vi "UpdateConfigInInternal.vi"(2 "error in (no error)":errorcluster, 3 "IntTime":i32, 4 "Instruments in":refnum<class "Instruments.lvclass">) -> (0 "error out":errorcluster, 1 "Instruments out":refnum<class "Instruments.lvclass">)   [LabVIEW 2012, in "Instruments.lvclass"]
uses:
  Instruments.lvclass
  Instruments.lvclass/Instruments.ctl
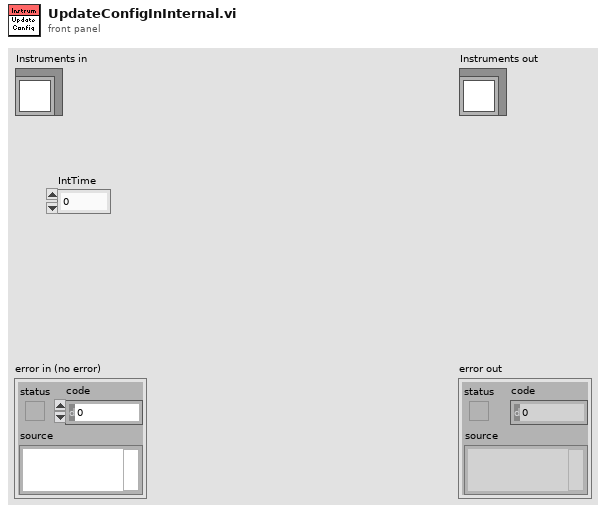
[diagram p1: front panel]
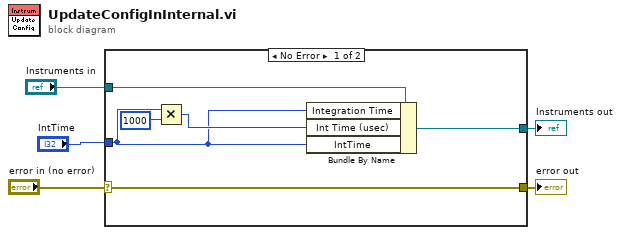
[diagram p0: block diagram]
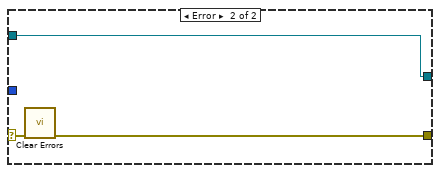
[diagram p2: hidden frame]
diagram:
  n1 = case shown="No Error" "error in (no error)" {
    selector: "error in (no error)" -> [w8 w13]
    tunnel: [w8 w12] -> w4
    tunnel: [w9 w14] -> w2
    tunnel: "Instruments in" -> [w7 w14]
    tunnel: "IntTime" -> [w6 _]
    frame No Error {
      n2 = Multiply(x=w6, y=1000) -> (x*y=w10:i32)
      n3 = Bundle By Name(cluster=w7, "Integration Time"=w6, "Int Time (usec)"=w10, "IntTime"=w6) -> (w9:refnum<class "Instruments.lvclass">)
    }
    frame Error {
      n4 = call <vilib>:"Clear Errors.vi"("error in (no error)"=w13) -> ("error out"=w12:errorcluster)  [unwired: 6 in]
    }
  }
  "error out" <- w4
  "Instruments out" <- w2
